vi "getMFC.vi"(11 "MFC ID Number":i32) -> (3 "MFC Input Cluster":T1 {"Flow (SCCM)" format="%#.6g"})   [LabVIEW 2011]
uses:
  GlobalVariables.vi
  Controls/MFC Cluster.ctl
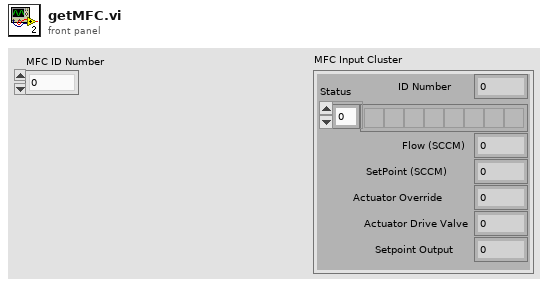
[diagram p1: front panel]
types:
  T1 = typedef "MFC Cluster.ctl" = cluster{"ID Number":u8, "Status":bool[], "Flow (SCCM)":dbl, "SetPoint (SCCM)":dbl, "Actuator Override":i8, "Actuator Drive Valve":i16, "Setpoint Output":dbl}
  T2 = typedef "Device Cluster.ctl" = cluster{"Dnet":string, "Node":i32, "Type":string, "ID Number":u8, "SCCM":dbl, "FullScale":dbl, "Input Bytes":i32, "Output Bytes":i32, "Input Start Location":i32, "Output Start Location":i32, "Enabled":bool, "Bytes":u8[]}
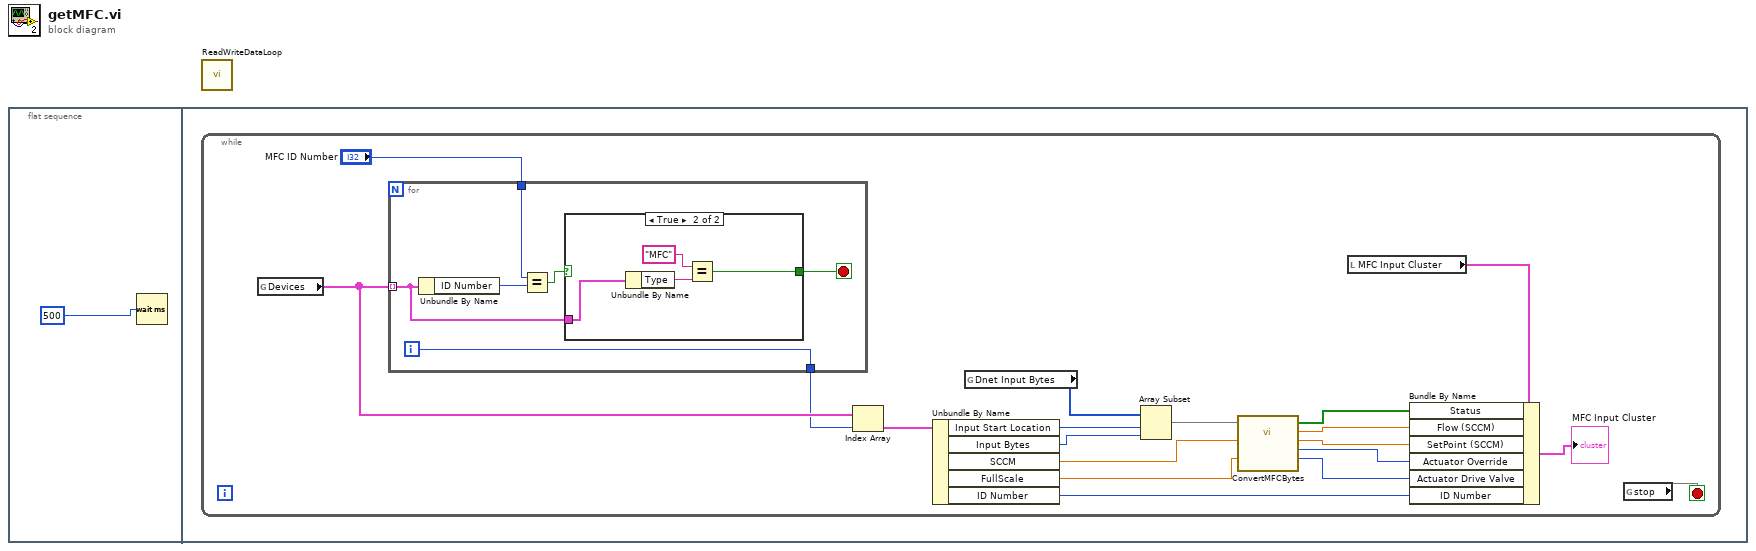
[diagram p0: block diagram]
diagram:
  n1 = flat-sequence {
    frame #0 {
      n2 = Wait (ms)(milliseconds to wait=500) -> ()  [unwired: 1 out]
    }
    frame #1 {
      n3 = while {
        stop <- w5 stop-if-true
        n4 = global read "GlobalVariables.vi" "Devices"() -> (w19:T2[])
        n5 = for {
          tunnel: w19 -> [w23] mode=indexing
          tunnel: "MFC ID Number" -> [w25]
          tunnel: [w21] -> w18
          i -> [w21]
          stop <- w22 stop-if-true
          n6 = Unbundle By Name(w23) -> ("ID Number"=w26:u8)
          n7 = Equal?(x=w25, y=w26) -> (x = y?=w24:bool)
          n8 = case shown="True" w24 {
            selector: w24 -> [w27 _]
            tunnel: w23 -> [_ w31]
            tunnel: [w27 w28] -> w22
            frame False {
            }
            frame True {
              n9 = Unbundle By Name(w31) -> ("Type"=w30:string)
              n10 = Equal?(x="MFC", y=w30) -> (x = y?=w28:bool)
            }
          }
        }
        n11 = Index Array(array=w19, index=w18) -> (element=w17:T2)
        n12 = Unbundle By Name(w17) -> ("Input Start Location"=w15:i32, "Input Bytes"=w14:i32, "SCCM"=w4:dbl, "FullScale"=w3:dbl, "ID Number"=w2:u8)
        n13 = global read "GlobalVariables.vi" "Dnet Input Bytes"() -> (w16:u8[])
        n14 = Array Subset(array=w16, index=w15, length=w14) -> (w11:u8[])
        n15 = call "ConvertMFCBytes.vi"("FullScale"=w3, "SCCM"=w4, "MFC Bytes"=w11) -> ("Actuator Drive Valve"=w7:i16, "Setpoint (SCCM)"=w8:dbl, "Flow (SCCM)"=w9:dbl, "Actuator Override"=w6:u8, "Status"=w10:bool[])  [unwired: 1 in]
        n16 = local read "MFC Input Cluster"() -> (w13:T1)
        n17 = Bundle By Name(cluster=w13, "Status"=w10, "Flow (SCCM)"=w9, "SetPoint (SCCM)"=w8, "Actuator Override"=w7, "Actuator Drive Valve"=w6, "ID Number"=w2) -> (→"MFC Input Cluster":T1)
        n18 = global read "GlobalVariables.vi" "stop"() -> (w5)
      }
    }
  }
  n19 = call "ReadWriteDataLoop.vi"() -> ()  [unwired: 11 in, 1 out]
